vi "test type.vi"() -> ()   [LabVIEW 2020]
uses:
  Nominal Client/Nominal Client.lvclass/Nominal Client.ctl
  nominal types/workspace/workspace.lvclass/workspace.ctl
  type/type.lvclass/type.ctl
  9b7bf359-1e3f-4ca3-8efc-68bf7bf3cf6b.vi
  f36276fe-c188-4252-be69-0cd9933e6484.vi
  type/name.set.vi
  type/name.get.vi
  type/createdAt.get.vi
  Nominal Client/private_data.set.vi
  nominal types/workspace/rid.get.vi
  nominal types/workspace/id.get.vi
  <vilib>/AdvancedString/1D String Array to Delimited String.vi
  Nominal Client/workspace.set.vi
  Nominal Client/http.put.vi
  type/name.set.vi/a9d8e627-8d17-4eab-b85a-f7c2878cfb23.vi
  Nominal Client/error.vi
  Nominal Client/trace.payload_sent.vi
  Nominal Client/trace.payload_received.vi
  Nominal Client/create.authorization_header.vi
  Nominal Client/error.vi/859f8e04-e495-489b-b5b4-7ac163f56130.vi
  Nominal Client/trace.calling_method.vi
  <vilib>/JDP Science/JDP Science Common Utilities/Trim Whitespace__JDP.vi
  Nominal Client/api_token.get.vi
  <vilib>/Utility/file.llb/Application Directory.vi
  <vilib>/Utility/error.llb/Error Cluster From Error Code.vi
  submodules/reqwest-labview/lv-src/reqwest/create.vi
  Nominal Client/Palette Items/who_am_i.vi
  Nominal Client/workspace_cache.get_from_rid.vi
  Nominal Client/workspace_cache.get.vi
  <vilib>/JDP Science/JSONtext/Variant to JSON Text.vi
  <vilib>/Utility/libraryn.llb/Get File Extension.vi
  Nominal Client/log_file.write.vi
  submodules/reqwest-labview/lv-src/reqwest/put.vi
  <vilib>/JDP Science/JSONtext/Get all Object Items.vi
  <vilib>/JDP Science/JSONtext/JSON text to Variant.vi
  type/type.from_json.vi
  User/User.lvclass
  Nominal Client/Nominal Client.lvclass
  nominal types/workspace/workspace.lvclass
  submodules/reqwest-labview/lv-src/reqwest/reqwest.lvclass
  <vilib>/JDP Science/JSONtext/LVClass Serializer/JSONtext LVClass Serializer.lvclass
  type/type.lvclass
panel:
  out "createdAt":timestamp
  in  "name 2":string
  out "name":string
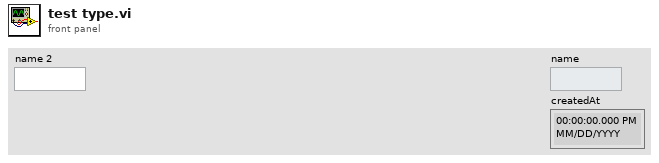
[diagram p1: front panel]
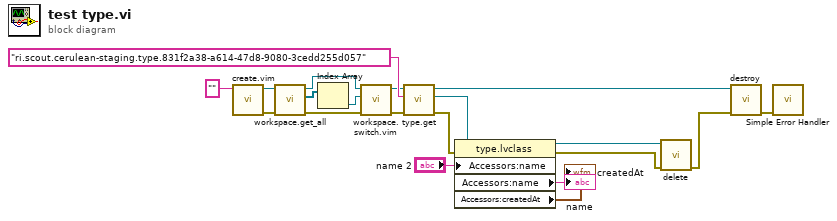
[diagram p0: block diagram]
diagram:
  n1 = call "create.vim"("API Token (string or path)"="") -> ("error out"=w13:errorcluster, "Nominal Client"=w14:refnum<class "Nominal Client.lvclass">)  [unwired: 8 in, 1 out]
  n2 = call "workspace.get_all.vi"("error in"=w13, "Nominal Client in"=w14) -> ("error out"=w16:errorcluster, "Workspaces"=w17:refnum<class "workspace.lvclass">[], "Nominal Client out"=w18:refnum<class "Nominal Client.lvclass">)  [unwired: 7 in]
  n3 = Index Array(array=w17) -> (element=w15:refnum<class "workspace.lvclass">)  [unwired: 1 in]
  n4 = call "workspace.switch.vim"("error in"=w16, "Workspace (Object, RID, Path)"=w15, "Nominal Client in"=w18) -> ("error out"=w10:errorcluster, "Nominal Client out"=w11:refnum<class "Nominal Client.lvclass">)  [unwired: 7 in]
  n5 = call "type.get.vi"("error in"=w10, "Type RID"="ri.scout.cerulean-staging.type.831f2a38-a614-47d8-9080-3cedd255d057" ("API Token (string or path)"), "Nominal Client in"=w11) -> ("error out"=w5:errorcluster, "type"=w8:refnum<class "type.lvclass">, "Nominal Client out"=w9:refnum<class "Nominal Client.lvclass">)  [unwired: 6 in]
  n6 = property class="type.lvclass"(reference=w8, error in=w5, "Accessors:name"="name 2") -> (reference out=w3:refnum<class "type.lvclass">, error out=w2:errorcluster, "Accessors:name"=→"name":string, "Accessors:createdAt"=→"createdAt":timestamp)
  n7 = call "delete.vi"("error in"=w2, "type in"=w3) -> ("error out"=w1:errorcluster)  [unwired: 8 in, 1 out]
  n8 = call "destroy.vi"("error in"=w1, "Nominal Client"=w9) -> ("error out"=w19:errorcluster)  [unwired: 9 in]
  n9 = call <vilib>:"Simple Error Handler.vi"("error in (no error)"=w19) -> ()  [unwired: 4 in, 5 out]
